vi "Teleop - Value Change Check (SubVI).vi"(9 "Shooter F":dbl, 10 "Shooter D":dbl, 11 "Shooter P":dbl) -> (1 "F Changed?":bool, 2 "D Changed?":bool, 3 "P Changed?":bool)   [LabVIEW 2019]
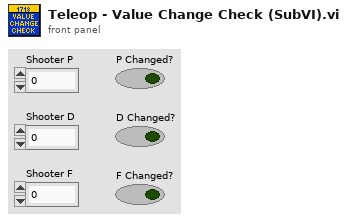
[diagram p1: front panel]
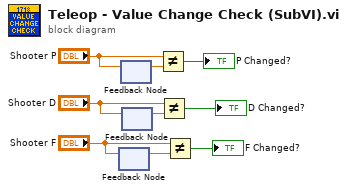
[diagram p0: block diagram]
diagram:
  n1 = feedback #1() -> (w4:dbl)  [unwired: 1 in]
  n2 = feedback-in #1("Shooter F") -> ()
  n3 = feedback #2() -> (w1:dbl)  [unwired: 1 in]
  n4 = feedback-in #2("Shooter P") -> ()
  n5 = feedback #3() -> (w7:dbl)  [unwired: 1 in]
  n6 = feedback-in #3("Shooter D") -> ()
  n7 = Not Equal?(x="Shooter P", y=w1) -> (x != y?=→"P Changed?":bool)
  n8 = Not Equal?(x="Shooter D", y=w7) -> (x != y?=→"D Changed?":bool)
  n9 = Not Equal?(x="Shooter F", y=w4) -> (x != y?=→"F Changed?":bool)
